vi "Read EIP Tag UUID.vi"(8 "error in":errorcluster, 11 "EIP Tags Channel in":refnum<class "EIP Tags Channel.lvclass">) -> (0 "error out":errorcluster, 2 "Tag Name":string, 3 "EIP Tags Channel out":refnum<class "EIP Tags Channel.lvclass">)   [LabVIEW 2013, in "EIP Tags Channel.lvclass"]
uses:
  EIP Tags Channel.lvclass
  EIP Tags Channel.lvclass/EIP Tags Channel.ctl
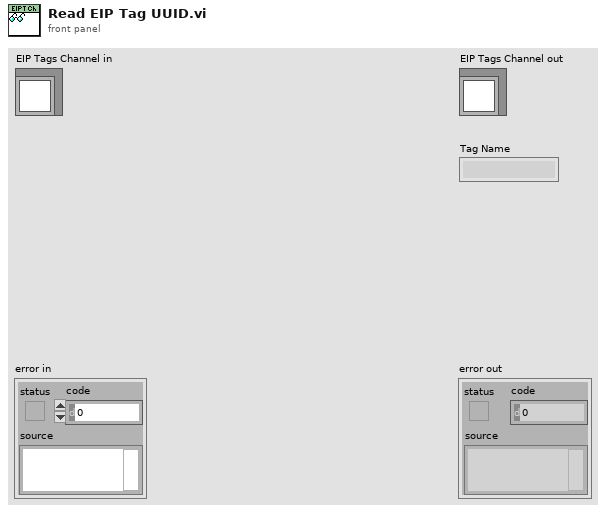
[diagram p1: front panel]
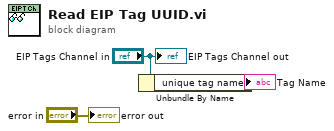
[diagram p0: block diagram]
diagram:
  n1 = Unbundle By Name("EIP Tags Channel in") -> ("unique tag name"=→"Tag Name":string)
  "error out" <- "error in"
  "EIP Tags Channel out" <- "EIP Tags Channel in"
